vi "myRIO_BRig_RT_dataTrial_ENL1_n.vi"() -> (2 "output_ENL1_n":i32)   [LabVIEW 2014]
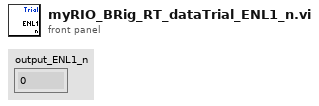
[diagram p1: front panel]
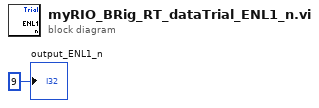
[diagram p0: block diagram]
diagram:
  "output_ENL1_n" <- 9 ("output_iBlock")
